vi "Launch RT Acq.vi"(5 "DO":T1[](array[typedef]), 7 "DI":T1[](array[typedef]), 8 "error in":errorcluster, 9 "AI":T4[](array[typedef]) {"Interface Data"."Timing"."sample mode" items=["Finite Samples"=10178, "Continuous Samples"=10123, "Hardware Timed Single Point"=12522]}, 10 "HW-IP":string[](array[string]), 11 "HW-Name":string[](array[string])) -> (0 "error out":errorcluster)   [LabVIEW 2021, in "Host Main.lvlib"]
doc: "This request event will launch the RT Acquisition module's based on the Given Input's.\n_____\nCreated using DQMH Event Scripter 7.0.1.1316."
uses:
  Host Main.lvlib
  Analog Output/Controls/AO JSON Data Cluster.ctl
  Analog Output/Controls/AO Interface Data Cluster.ctl
  Analog Output/Controls/AO Channel Configuration Cluster.ctl
  Analog Output/Controls/AO Timing Cluster.ctl
  Digital Output/Controls/DIO Configuration cluster.ctl
  Digital Output/Controls/DIO Interface Data.ctl
  Digital Output/SubVIs/Digital Dynamic Cluster.ctl
  Launch RT Acq Argument--cluster.ctl
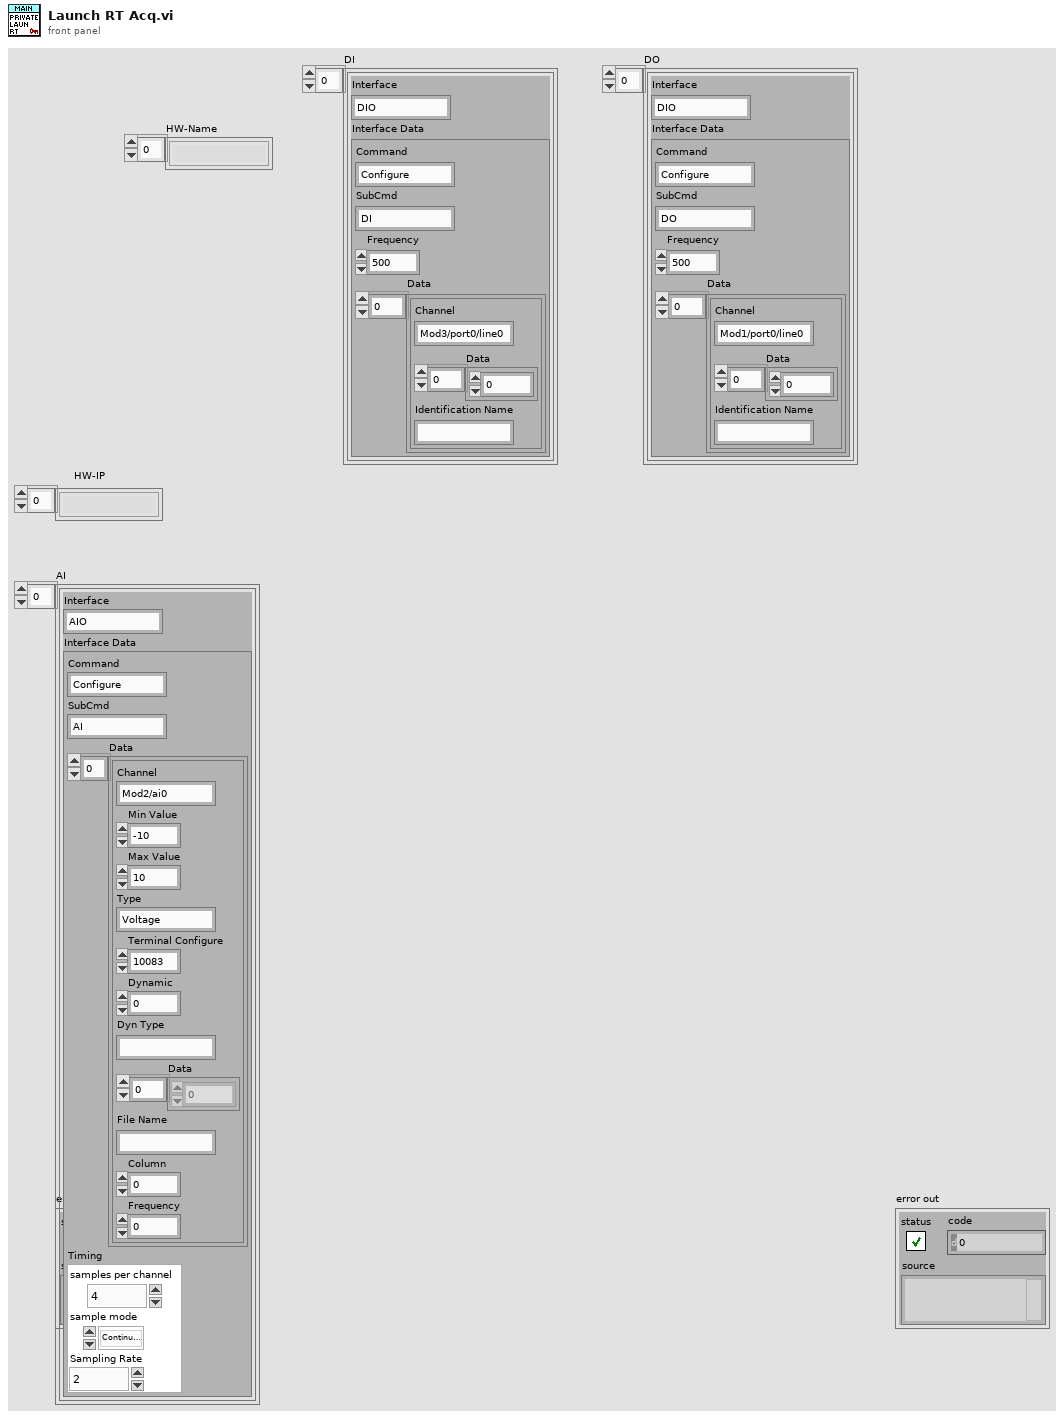
[diagram p1: front panel]
types:
  T1 = typedef "DIO Configuration cluster.ctl" = cluster{"Interface":string, "Interface Data":T2}
  T2 = typedef "DIO Interface Data.ctl" = cluster{"Command":string, "SubCmd":string, "Frequency":u16, "Data":T3[]}
  T3 = typedef "Digital Dynamic Cluster.ctl" = cluster{"Channel":string, "Data":u8[], "Identification Name":string}
  T4 = typedef "AO JSON Data Cluster.ctl" = cluster{"Interface":string, "Interface Data":T5}
  T5 = typedef "AO Interface Data Cluster.ctl" = cluster{"Command":string, "SubCmd":string, "Data":T6[], "Timing":T7}
  T6 = typedef "AO Channel Configuration Cluster.ctl" = cluster{"Channel":string, "Min Value":dbl, "Max Value":dbl, "Type":string, "Terminal Configure":u16, "Dynamic":u8, "Dyn Type":string, "Data":dbl[], "File Name":string, "Column":i32, "Frequency":dbl}
  T7 = typedef "AO Timing Cluster.ctl" = cluster{"samples per channel":i32, "sample mode":i32, "Sampling Rate":dbl}
  T8 = typedef "Host Main.lvlib/Launch RT Acq Argument--cluster.ctl" = cluster{"HW-IP":string[], "HW-Name":string[], "AI":T4[], "DI":T1[], "DO":T1[]}
  T9 = typedef "Host Main.lvlib/Request Events--cluster.ctl" = cluster{"Show Panel":refnum<user-event>, "Hide Panel":refnum<user-event>, "Get Module Execution Status":refnum<user-event>, "Show Diagram":refnum<user-event>, "Private":cluster{"Launch RT Acq":refnum<user-event>}, "Stop Module":refnum<user-event>, "Launch TP":refnum<user-event>}
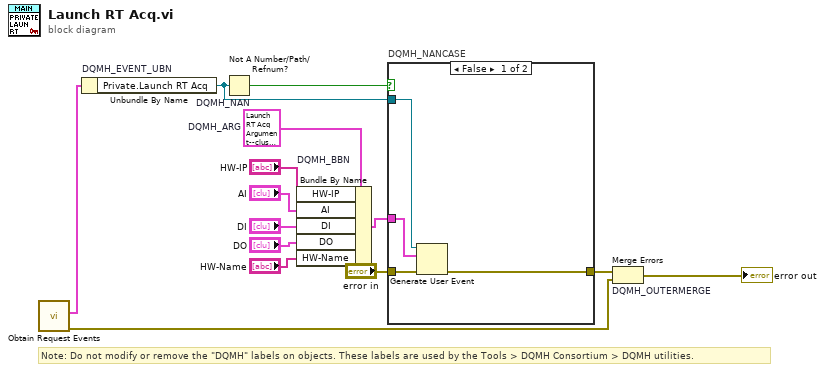
[diagram p0: block diagram]
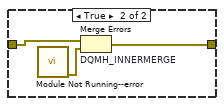
[diagram p2: hidden frame]
diagram:
  w8 = T8 data[24185B]  # DQMH_ARG
  # "Note: Do not modify or remove the \"DQMH\" labels on objects. These labels are used by the Tools > DQMH Consortium > DQMH utilities."
  n1 = call "Obtain Request Events.vi"() -> ("error out"=w3:errorcluster, "Host Main Request Events"=w2:T9)  [unwired: 10 in]
  n2 = Unbundle By Name "DQMH_EVENT_UBN"(w2) -> ("Private.Launch RT Acq"=w10:refnum<user-event>)
  n3 = Not A Number/Path/Refnum? "DQMH_NAN"(number/path/refnum=w10) -> (NaN/Path/Refnum?=w11:bool)
  n4 = Bundle By Name "DQMH_BBN"(cluster=w8, "HW-IP"="HW-IP", "AI"="AI", "DI"="DI", "DO"="DO", "HW-Name"="HW-Name") -> (w12:T8)
  n5 = case "DQMH_NANCASE" shown="False" w11 {
    tunnel: "error in" -> [w18 w21]
    tunnel: [w17 w20] -> w9
    tunnel: w10 -> [w16 _]
    tunnel: w12 -> [w15 _]
    frame False {
      n6 = Generate User Event(user event=w16, event data cluster=w15, error in=w18) -> (error out=w17:errorcluster)  [unwired: 1 in, 1 out]
    }
    frame True {
      n7 = call "Module Not Running--error.vi"() -> ("error out"=w19:errorcluster)  [unwired: 11 in]
      n8 = Merge Errors "DQMH_INNERMERGE"(w21, w19) -> (w20:errorcluster)
    }
  }
  n9 = Merge Errors "DQMH_OUTERMERGE"(w9, w3) -> (→"error out":errorcluster)
